vi "Shutdown.vi"(8 "Error In":errorcluster, 11 "Context In":refnum<class "Context.lvclass">) -> (0 "Error Out":errorcluster, 2 "Data":refnum<class "Datum.lvclass">, 3 "Context Out":refnum<class "Context.lvclass">)   [LabVIEW 2018, in "Toolkit.lvlib" / "Context.lvclass"]
uses:
  Context.lvclass
  Data/Datum/Datum.lvclass
  Context.lvclass/Context.ctl
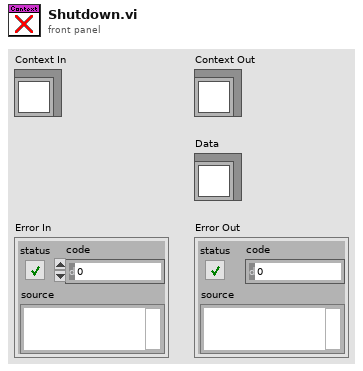
[diagram p1: front panel]
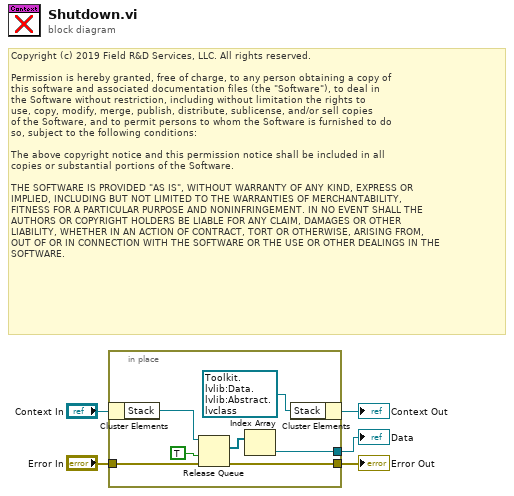
[diagram p0: block diagram]
diagram:
  # "Copyright (c) 2019 Field R&D Services, LLC. All rights reserved.\n\nPermission is hereby granted, free of charge, to any person obtaining a copy of\nthis software and associated documentation files (the \"Software\"), to deal in\nthe Software without restriction, including without limitation the rights to\nuse, copy, modify, merge, publish, distribute, sublicense, and/or sell copies\nof the Software, and to permit persons to whom the Software is furnished to do\nso, subject to the following conditions:\n\nThe above copyright notice and this permission notice shall be included in all\ncopies or substantial portions of the Software.\n\nTHE SOFTWARE IS PROVIDED \"AS IS\", WITHOUT WARRANTY OF ANY KIND, EXPRESS OR\nIMPLIED, INCLUDING BUT NOT LIMITED TO THE WARRANTIES OF MERCHANTABILITY,\nFITNESS FOR A PARTICULAR PURPOSE AND NONINFRINGEMENT. IN NO EVENT SHALL THE\nAUTHORS OR COPYRIGHT HOLDERS BE LIABLE FOR ANY CLAIM, DAMAGES OR OTHER\nLIABILITY, WHETHER IN AN ACTION OF CONTRACT, TORT OR OTHERWISE, ARISING FROM,\nOUT OF OR IN CONNECTION WITH THE SOFTWARE OR THE USE OR OTHER DEALINGS IN THE\nSOFTWARE."
  n1 = in-place {
    in-place-border: "Error In" -> [w11]
    in-place-border: [w10] -> w4
    in-place-border: [w6] -> w1
    n2 = in-place-cluster #1("Context In") -> ("Stack"=w9:refnum<queue>)
    n3 = Release Queue(queue=w9, force destroy? (F)=TRUE, error in (no error)=w11) -> (remaining elements=w7:refnum<class "Datum.lvclass">[], error out=w10:errorcluster)  [unwired: 1 out]
    n4 = Index Array(array=w7) -> (element=w6:refnum<class "Datum.lvclass">)  [unwired: 1 in]
    n5 = in-place-cluster #1("Stack"=refnum<queue> refnum) -> (→"Context Out":refnum<class "Context.lvclass">)
  }
  "Error Out" <- w4
  "Data" <- w1
